vi "001 escriure a fitxer.vi"() -> ()   [LabVIEW 2019]
uses:
  <vilib>/Analysis/baseanly.llb/Mean (DBL).vi
  <vilib>/Analysis/NI_AALBase.lvlib
panel:
  out "min value":dbl
  out "max index(es)":i32
  out "mean":dbl format="%0.2f"
  out "Waveform Chart":dbl(graph)
  in  "stop":bool
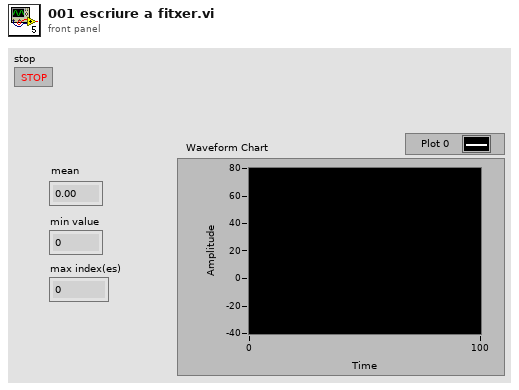
[diagram p1: front panel]
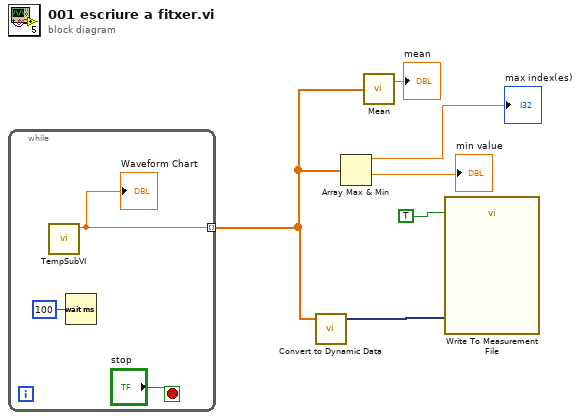
[diagram p0: block diagram]
diagram:
  n1 = while {
    tunnel: [w7] -> w4 mode=indexing
    stop <- "stop" stop-if-true
    n2 = call "TempSubVI.vi"() -> ("temp"=w7:dbl)  [unwired: 11 in]
    "Waveform Chart" <- w7
    n3 = Wait (ms)(milliseconds to wait=u32 100) -> ()  [unwired: 1 out]
  }
  n4 = call "Convert to Dynamic Data"("Array"=w4) -> ("Dynamic Data Type"=w6:dynamicdata)  [unwired: 3 in]
  n5 = Array Max & Min(array=w4) -> (max value=→"max index(es)":dbl, min value=→"min value":dbl)  [unwired: 2 out]
  n6 = call-poly <vilib>:"Mean.vi"("X"=w4) -> ("mean"=→"mean":dbl)  [unwired: 1 out]
  n7 = call "Write To Measurement File"("Signals"=w6, "Reset"=TRUE) -> ()  [unwired: 15 in, 3 out]
